vi "Get Instrument Config Filepath.vi"(8 "error in":errorcluster, 11 "Sequence Context In":refnum<k7>) -> (0 "error out":errorcluster, 2 "File Path":path, 3 "Sequence Context out":refnum<k7>)   [LabVIEW 2023, in "Instrument Config.lvlib"]
uses:
  Instrument Config.lvlib
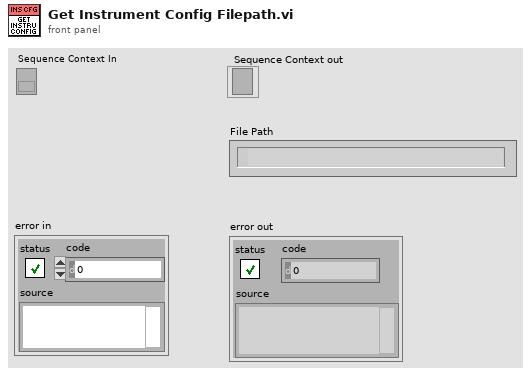
[diagram p1: front panel]
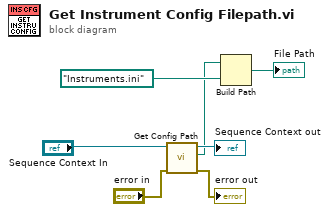
[diagram p0: block diagram]
diagram:
  n1 = call "Get Config Path.vi"("error in"="error in", "Sequence Context In"="Sequence Context In") -> ("error out"=→"error out":errorcluster, "Configuration Path"=w2:path, "Sequence Context out"=→"Sequence Context out":refnum<k7>)  [unwired: 7 in]
  n2 = Build Path(base path=w2, name or relative path=path "Instruments.ini") -> (appended path=→"File Path":path)
